vi "Function_Find Circle #.vi"(8 "Error in":errorcluster, 9 "CoordSys In":T1 {"Measurement System"."Axis Reference" items=["Direct", "Indirect"]; "Measurement System"."Angle (deg)" format="%.2f"; "Measurement System"."Origin"."Y" format="%.2f"; "Measurement System"."Origin"."X" format="%.2f"; "Reference System"."Axis Reference" items=["Direct", "Indirect"]; "Reference System"."Angle (deg)" format="%.2f"; "Reference System"."Origin"."Y" format="%.2f"; "Reference System"."Origin"."X" format="%.2f"}, 10 "Data Cluster In":cluster{"Name":string, "Variant In":variant}, 11 "Image Src":T2) -> (0 "Error Out":errorcluster, 3 "Circle Center":cluster{"X":sgl, "Y":sgl} {"Y" format="%.2g"; "X" format="%.2f"})   [LabVIEW 2013]
uses:
  <vilib>/vision/Image Controls.llb/IMAQ Image.ctl
  Control/Control Find Circle.ctl
  <vilib>/vision/Measure.llb/Edge Options.ctl
  <vilib>/vision/Measure.llb/Edge Polarity.ctl
  <vilib>/vision/NI_Vision_Development_Module.lvlib
  <vilib>/gmath/NI_Gmath.lvlib
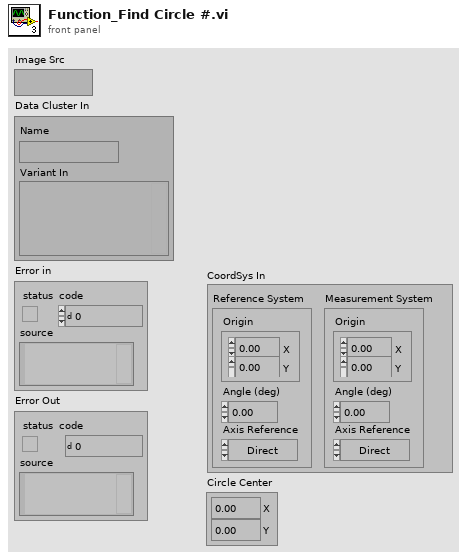
[diagram p1: front panel]
types:
  T1 = typedef "IMAQ Coordinate System" = cluster{"Reference System":cluster{"Origin":cluster{"X":sgl, "Y":sgl}, "Angle (deg)":sgl, "Axis Reference":u32}, "Measurement System":cluster{"Origin":cluster{"X":sgl, "Y":sgl}, "Angle (deg)":sgl, "Axis Reference":u32}}
  T2 = typedef "IMAQ Image.ctl" = refnum<image>
  T3 = typedef "Control Find Circle.ctl" = cluster{"ROI Descriptor":cluster{"Global Rectangle":i32[], "Contours":cluster{"ID":enum32{"External", "Internal"}, "Type":u32, "Coordinates":i32[]}[]}, "Step Size":dbl, "Scan Direction":u16, "Edge Options":T4}
  T4 = typedef "Edge Options.ctl" = cluster{"Edge Polarity":T5, "Kernel Size":u32, "Width":u32, "Minimum Edge Strength":sgl, "Interpolation Type":enum32{"Zero Order", "Bilinear", "Quadratic", "Cubic", "Bilinear Fixed"}, "Data Processing Method":enum32{"Average", "Median"}}
  T5 = typedef "Edge Polarity.ctl" = u32
  T6 = enum16{"Get First Edge", "Get First + Last Edge", "Get All Edges", "Get Best Edge"}
  T7 = cluster{"Global Rectangle":i32[], "Contours":cluster{"ID":enum32{"External", "Internal"}, "Type":u32, "Coordinates":i32[]}[]}
  T8 = cluster{"Origin":cluster{"X":sgl, "Y":sgl}, "Angle (deg)":sgl, "Axis Reference":u32}
  T9 = typedef "ROI Descriptor" = cluster{"Global Rectangle":i32[], "Contours":cluster{"ID":enum32{"External", "Internal"}, "Type":u32, "Coordinates":i32[]}[]}
  T10 = typedef "Edge New.ctl" = cluster{"Location (Pixel)":cluster{"X":sgl, "Y":sgl}, "Location (Real-World)":cluster{"X":sgl, "Y":sgl}, "Distance (Pixel)":dbl, "Distance (Real-World)":dbl, "Strength":dbl, "Noise":dbl, "Rising?":bool}
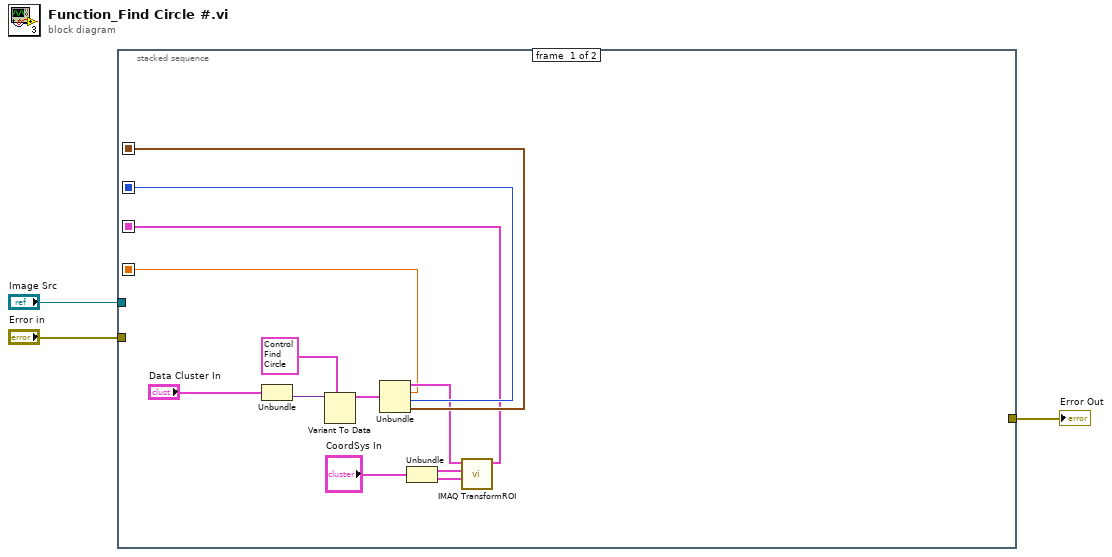
[diagram p0: block diagram]
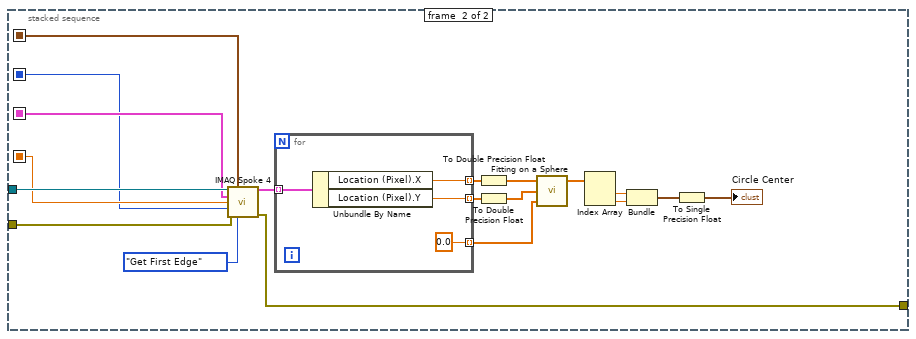
[diagram p2: hidden frame]
diagram:
  n1 = stacked-sequence {
    seq-local: [w6 _] -> [_ w17]
    seq-local: [w11 _] -> [_ w16]
    seq-local: [w10 _] -> [_ w19]
    seq-local: [w4 _] -> [_ w18]
    tunnel: "Error in" -> [_ w21]
    tunnel: "Image Src" -> [_ w23]
    tunnel: [_ w20] -> w1
    frame #0 {
      n2 = Unbundle("Data Cluster In") -> ("Variant In"=w14:variant)  [unwired: 1 out]
      n3 = Variant To Data(type=T3 {"ROI Descriptor"={"Global Rectangle"=[], "Contours"=[]}, "Step Size"=0.0, "Scan Direction"=5, "Edge Options"={"Edge Polarity"=0, "Kernel Size"=0, "Width"=0, "Minimum Edge Strength"=0.0, "Interpolation Type"=enum."Zero Order", "Data Processing Method"=enum."Average"}} ("蛾み_Setting"), Variant=w14) -> (data=w13:T3)  [unwired: 1 in, 1 out]
      n4 = Unbundle(w13) -> ("ROI Descriptor"=w5:T7, "Step Size"=w4:dbl, "Scan Direction"=w11:u16, "Edge Options"=w10:T4)
      n5 = Unbundle("CoordSys In") -> ("Reference System"=w8:T8, "Measurement System"=w7:T8)
      n6 = call "IMAQ TransformROI"("New Reference"=w7, "Base Reference"=w8, "ROI Descriptor"=w5) -> ("ROI Descriptor out"=w6:T9)  [unwired: 7 in, 1 out]
    }
    frame #1 {
      n7 = call "IMAQ Spoke 4"("Image"=w23, "Edge Options"=w19, "ROI Descriptor"=w17, "Step Size"=w18, "Scan Direction"=w16, "error in (no error)"=w21, "Process"=T6."Get First Edge") -> ("First Edges"=w26:T10[], "error out"=w20:errorcluster)  [unwired: 5 in, 2 out]
      n8 = for {
        tunnel: w26 -> [w38] mode=indexing
        tunnel: [w37] -> w24 mode=indexing
        tunnel: [w36] -> w25 mode=indexing
        tunnel: [0.0] -> w29 mode=indexing
        n9 = Unbundle By Name(w38) -> ("Location (Pixel).X"=w37:sgl, "Location (Pixel).Y"=w36:sgl)
      }
      n10 = To Double Precision Float(number=w24) -> (double precision float=w27:dbl[])
      n11 = To Double Precision Float(number=w25) -> (double precision float=w28:dbl[])
      n12 = call <vilib>:"Fitting on a Sphere.vi"("Z"=w29, "Y"=w28, "X"=w27) -> ("x0, y0, z0"=w30:dbl[])  [unwired: 2 out]
      n13 = Index Array(array=w30) -> (element #1=w31:dbl, element #2=w32:dbl)  [unwired: 2 in]
      n14 = Bundle(w31, w32) -> (w33:cluster{dbl, dbl})  [unwired: 1 in]
      n15 = To Single Precision Float(number=w33) -> (single precision float=→"Circle Center":cluster{sgl, sgl})
    }
  }
  "Error Out" <- w1
